vi "בדיקת מתח תפיסה של סליל פיקוד ללא עומס Mod.vi"(8 "error":errorcluster, 9 "מתח מקס":dbl=18.0 format="%#_13g", 10 "שם הממסר":string="0410-24534 15A ממסר", 11 "Path for Log":path) -> (0 "error out":errorcluster, 1 "מצב ממסר פתוח/סגור":bool, 2 "מתח סגירת הממסר":dbl format="%.4f", 3 "מתח מוצא מהספק":dbl format="%.4f", 5 "resultUserPrompt":bool)   [LabVIEW 2014]
uses:
  <vilib>/DAQmx/create/channels.llb/DAQmx Create Channel (DO-Digital Output).vi
  <vilib>/DAQmx/write.llb/DAQmx Write (Digital Bool 1Line 1Point).vi
panel:
  out "progress":dbl(slide) scale=0.0..36.0
  out "error IO DMM":errorcluster
  in  "Stop Button":bool
  # "Right-Click to\nexplain error"
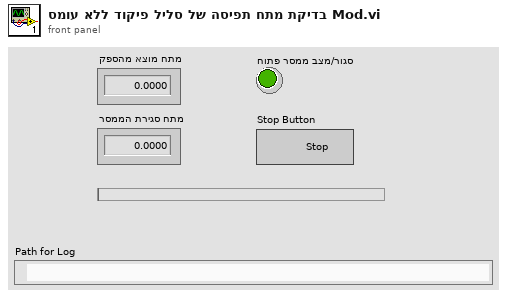
[diagram p1: front panel]
types:
  T1 = enum32{"Invalid", "Standard", "Closed", "Hidden", "Minimized", "Maximized"}
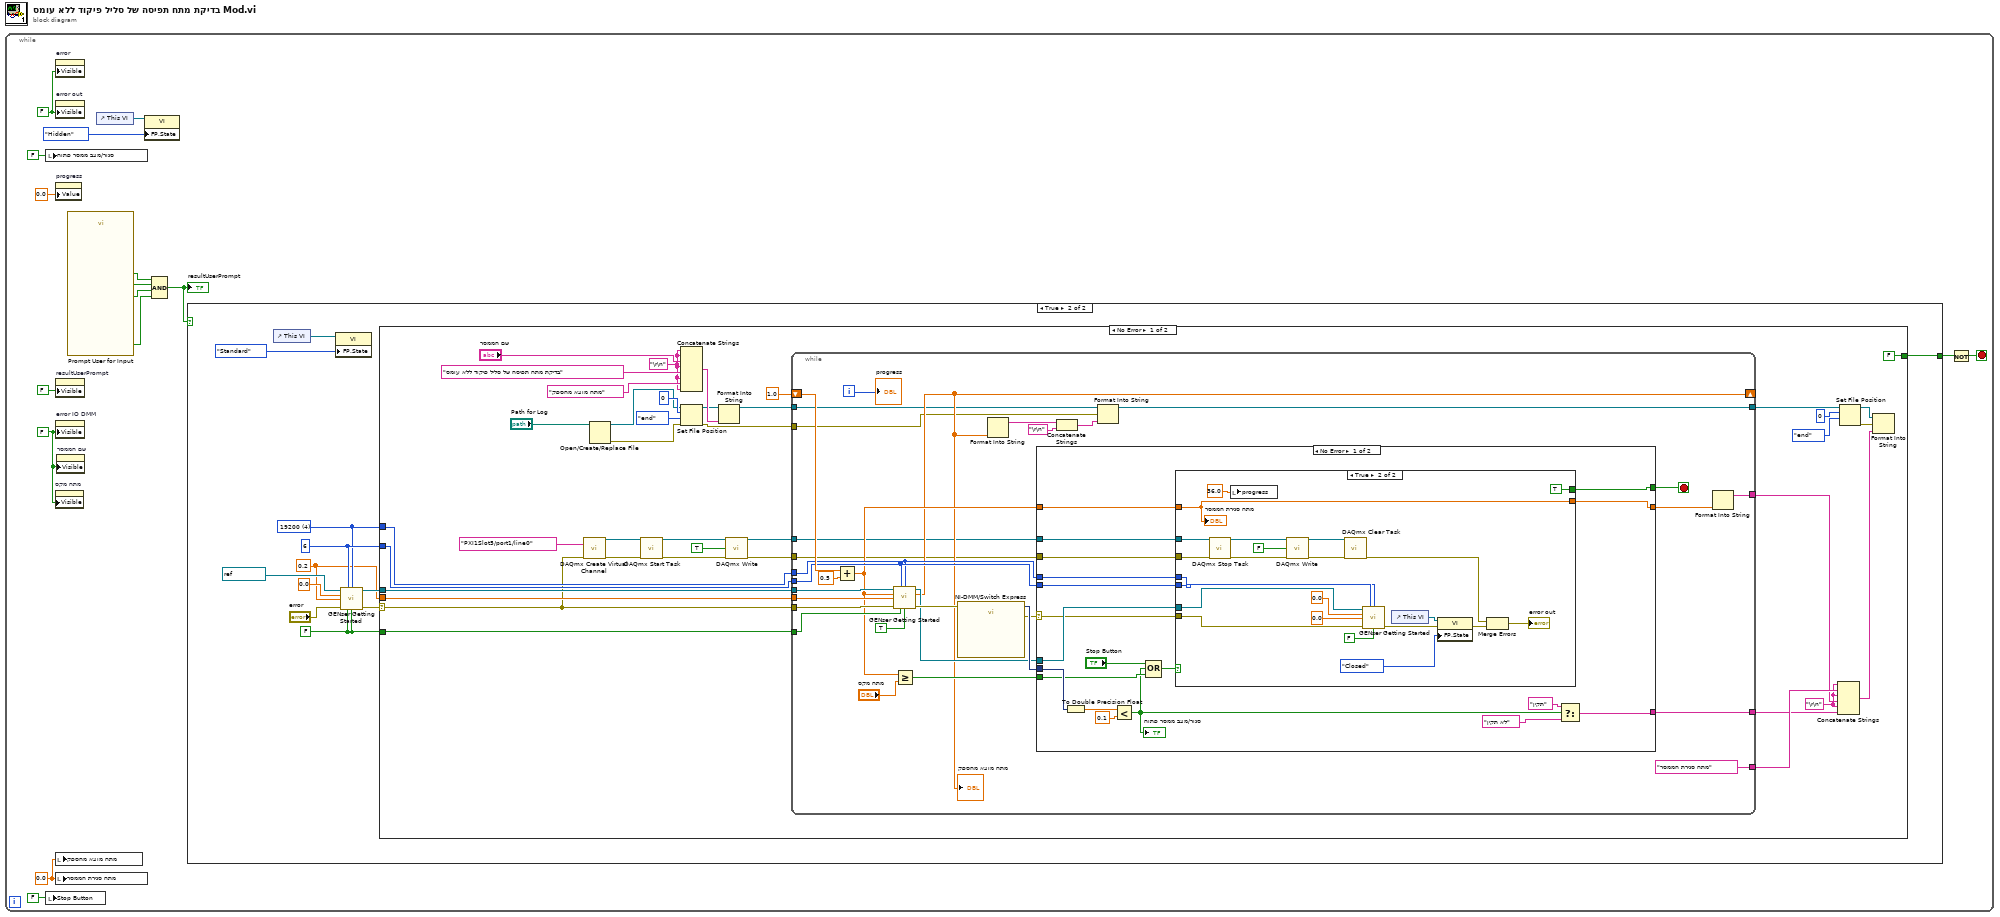
[diagram p0: block diagram]
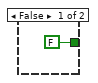
[diagram p2: hidden frame]
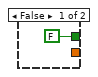
[diagram p3: hidden frame]
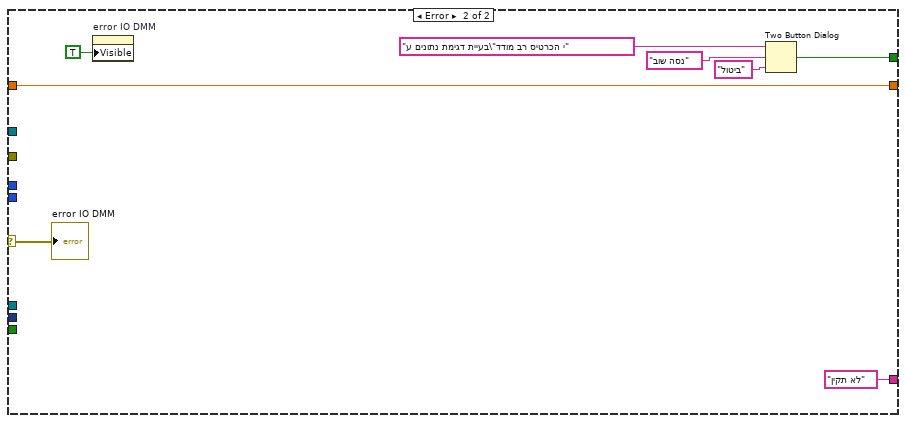
[diagram p4: hidden frame]
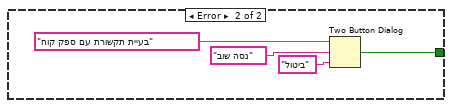
[diagram p5: hidden frame]
diagram:
  n1 = while {
    stop <- w4 stop-if-true
    w3 = FALSE ("Visible")
    w9 = 0.0 ("signals out")
    w1 = FALSE ("Visible")
    n2 = local write "מצב ממסר פתוח/סגור"(FALSE ("מגע סגור")) -> ()
    n3 = local write "Stop Button"(FALSE ("Reset (T)")) -> ()
    n4 = property on="מתח מקס" class="DigNum (strict)"("Visible"=w1) -> ()  [unwired: 2 in, 2 out]
    n5 = property on="error" class="Clust (strict)"("Visible"=w3) -> ()  [unwired: 2 in, 2 out]
    n6 = property on="error out" class="Clust (strict)"("Visible"=w3) -> ()  [unwired: 2 in, 2 out]
    n7 = property on="progress" class="Slide (strict)"("Value"=0.0 ("progress")) -> ()  [unwired: 2 in, 2 out]
    n8 = property on="resultUserPrompt" class="Bool (strict)"("Visible"=FALSE) -> ()  [unwired: 2 in, 2 out]
    n9 = property on="error IO DMM" class="Clust (strict)"("Visible"=w1) -> ()  [unwired: 2 in, 2 out]
    n10 = local write "מתח מוצא מהספק"(w9) -> ()
    n11 = local write "מתח סגירת הממסר"(w9) -> ()
    n12 = property on="שם הממסר" class="Str"("Visible"=w1) -> ()  [unwired: 2 in, 2 out]
    n13 = call "Prompt User for Input"() -> ("הדקי הרב מודד"=w7:bool, "מגע שלילי"=w13:bool, "מגע חיובי"=w14:bool, "OK"=w8:bool)  [unwired: 15 in, 1 out]
    n14 = control-ref of="This VI"() -> (w6:refnum<vi>)
    n15 = property class="VI"(reference=w6, "FP.State"=T1."Hidden" ("Front Panel Window:State")) -> ()  [unwired: 1 in, 2 out]
    n16 = Compound Arithmetic op=AND(w8, w14, w13, w7) -> (w15:bool)
    "resultUserPrompt" <- w15
    n17 = case shown="True" w15 {
      tunnel: [FALSE ("T button?") w23] -> w16
      frame False {
      }
      frame True {
        w22 = FALSE ("Output On (T)")
        w27 = u16 4 items=["1200", "2400", "4800", "9600", "19200"] ("BAUD")
        w28 = i16 6 ("GEN Addr")
        w24 = 0.2 ("Current Limit")
        n18 = control-ref of="This VI"() -> (w20:refnum<vi>)
        n19 = property class="VI"(reference=w20, "FP.State"=T1."Standard" ("Front Panel Window:State")) -> ()  [unwired: 1 in, 2 out]
        n20 = call "GENser Getting Started.vi"("VISA"=refnum<visa-resource-name> "COM6", "GEN Addr"=w28, "BAUD"=w27, "Voltage Limit"=0.0, "Current Limit"=w24, "error"="error", "Reset (T)"=w22, "Output On (T)"=w22) -> ("VISA out"=w29:refnum<visa-resource-name>, "error out"=w19:errorcluster)  [unwired: 4 in, 2 out]
        n21 = case shown="No Error" w19 {
          selector: w19 -> [w30 _]
          tunnel: w29 -> [w68 _]
          tunnel: w28 -> [w67 _]
          tunnel: w27 -> [w66 _]
          tunnel: w22 -> [w65 _]
          tunnel: w24 -> [w64 _]
          tunnel: [FALSE w151] -> w23
          frame No Error {
            w39 = "\r\n"
            w58 = "\r\n"
            n22 = call-poly <vilib>:"DAQmx Create Virtual Channel.vi"("lines"=tag "PXI1Slot5/port1/line0", "error in"=w30) -> ("task out"=w37:refnum<k21>, "error out"=w38:errorcluster)  [unwired: 12 in]
            n23 = Open/Create/Replace File(file path (use dialog)="Path for Log") -> (refnum out=w49:refnum<file>, error out=w48:errorcluster)  [unwired: 5 in, 1 out]
            n24 = call <vilib>:"DAQmx Start Task.vi"("task/channels in"=w37, "error in"=w38) -> ("task out"=w34:refnum<k21>, "error out"=w33:errorcluster)  [unwired: 12 in]
            n25 = Concatenate Strings(w39, w39, "שם הממסר", w39, "בדיקת מתח תפיסה של סליל פיקוד ללא עומס", w39, "מתח מוצא מהספק", w39) -> (w45:string)
            n26 = Set File Position(offset (in bytes) (0)=i64 0, refnum=w49, from (0:start)=enum16{"start", "end", "current"}."end", error in=w48) -> (refnum out=w41:refnum<file>, error out=w46:errorcluster)
            n27 = Format Into String(initial string=w41, w45) -> (resulting string=w40:refnum<file>)  [unwired: 2 in, 1 out]
            n28 = call-poly <vilib>:"DAQmx Write.vi"("task/channels in"=w34, "data"=TRUE, "error in"=w33) -> ("task out"=w32:refnum<k21>, "error out"=w31:errorcluster)  [unwired: 10 in, 1 out]
            n29 = while {
              tunnel: w68 -> [w88]
              tunnel: w30 -> [w99]
              tunnel: w67 -> [w90]
              tunnel: w66 -> [w89]
              tunnel: w65 -> [w98]
              tunnel: w64 -> [w96]
              shift-right: [w80] -> _
              shift-left: 1.0 ("y") -> [w94]
              tunnel: ["מתח סגירת הממסר"] -> w61
              tunnel: [w78] -> w60
              tunnel: [w77] -> w59
              tunnel: [w74] -> w57
              tunnel: w40 -> [w73]
              tunnel: w46 -> [w72]
              tunnel: w32 -> [w70]
              tunnel: w31 -> [w69]
              i -> [w81]
              stop <- w91 stop-if-true
              n30 = Add(x=w94, y=0.5) -> (x+y=w82:dbl)
              n31 = call "GENser Getting Started.vi"("VISA"=w88, "GEN Addr"=w90, "BAUD"=w89, "Voltage Limit"=w82, "Current Limit"=w96, "error"=w99, "Reset (T)"=w98, "Output On (T)"=TRUE) -> ("VISA out"=w87:refnum<visa-resource-name>, "Output Voltage"=w80:dbl, "error out"=w93:errorcluster)  [unwired: 4 in, 1 out]
              "מתח מוצא מהספק" <- w80
              n32 = Greater Or Equal?(x=w82, y="מתח מקס") -> (x >= y?=w85:bool)
              n33 = call "NI-DMM/Switch Express"("error in"=w93) -> ("signals out"=w92:dynamicdata, "error out"=w84:errorcluster)  [unwired: 16 in, 1 out]
              n34 = Format Into String(w80) -> (resulting string=w75:string)  [unwired: 3 in, 1 out]
              n35 = case shown="No Error" w84 {
                selector: w84 -> [w110 w150]
                tunnel: w92 -> [w118 _]
                tunnel: [w107 w146] -> w91
                tunnel: w90 -> [w115 _]
                tunnel: w89 -> [w114 _]
                tunnel: w87 -> [w113 _]
                tunnel: w85 -> [w112 _]
                tunnel: w82 -> [w111 w144]
                tunnel: [w106 w144] -> w83
                tunnel: [w103 "לא תקין"] -> w77
                tunnel: w70 -> [w101 _]
                tunnel: w69 -> [w100 _]
                frame No Error {
                  n36 = To Double Precision Float(number=w118) -> (double precision float=w109:dbl)
                  n37 = Less?(x=w109, y=0.1) -> (x < y?=w102:bool)
                  "מצב ממסר פתוח/סגור" <- w102
                  n38 = Compound Arithmetic op=OR("Stop Button", w102, w112) -> (w117:bool)
                  n39 = case shown="True" w117 {
                    tunnel: [FALSE TRUE] -> w107
                    tunnel: w115 -> [_ w142]
                    tunnel: w114 -> [_ w141]
                    tunnel: w113 -> [_ w140]
                    tunnel: w110 -> [_ w137]
                    tunnel: w111 -> [_ w132]
                    tunnel: [_ w132] -> w106
                    tunnel: w101 -> [_ w122]
                    tunnel: w100 -> [_ w121]
                    frame False {
                    }
                    frame True {
                      n40 = call <vilib>:"DAQmx Stop Task.vi"("task/channels in"=w122, "error in"=w121) -> ("task out"=w130:refnum<k21>, "error out"=w128:errorcluster)  [unwired: 12 in]
                      n41 = local write "progress"(36.0 ("progress")) -> ()
                      n42 = call-poly <vilib>:"DAQmx Write.vi"("task/channels in"=w130, "data"=FALSE, "error in"=w128) -> ("task out"=w127:refnum<k21>, "error out"=w126:errorcluster)  [unwired: 10 in, 1 out]
                      n43 = call <vilib>:"DAQmx Clear Task.vi"("task in"=w127, "error in"=w126) -> ("error out"=w123:errorcluster)  [unwired: 13 in]
                      n44 = call "GENser Getting Started.vi"("VISA"=w140, "GEN Addr"=w142, "BAUD"=w141, "Voltage Limit"=0.0, "Current Limit"=0.0, "error"=w137, "Output On (T)"=FALSE) -> ("error out"=w120:errorcluster)  [unwired: 5 in, 3 out]
                      n45 = control-ref of="This VI"() -> (w134:refnum<vi>)
                      n46 = property class="VI"(reference=w134, error in=w120, "FP.State"=T1."Closed" ("Front Panel Window:State")) -> (error out=w124:errorcluster)  [unwired: 1 out]
                      n47 = Merge Errors(w123, w124) -> (→"error out":errorcluster)
                      "מתח סגירת הממסר" <- w132
                    }
                  }
                  n48 = Select(t="תקין", s=w102, f="לא תקין") -> (s? t:f=w103:string)
                }
                frame Error {
                  n49 = property on="error IO DMM" class="Clust (strict)"("Visible"=TRUE) -> ()  [unwired: 2 in, 2 out]
                  n50 = Two Button Dialog(message="בעיית דגימת נתונים ע\"י הכרטיס רב מודד", 1:"ביטול" ("F button name (\"Cancel\")"), 2:"נסה שוב" ("T button name (\"OK\")")) -> (T button?=w146:bool)
                  "error IO DMM" <- w150
                }
              }
              n51 = Concatenate Strings(w75, "\r\n") -> (w71:string)
              n52 = Format Into String(initial string=w73, error in=w72, w71) -> (resulting string=w74:refnum<file>)  [unwired: 1 in, 1 out]
              n53 = Format Into String(w83) -> (resulting string=w78:string)  [unwired: 3 in, 1 out]
              "progress" <- w81
            }
            n54 = Concatenate Strings(w58, w61, w58, w60, w58, w59) -> (w52:string)
            n55 = Set File Position(offset (in bytes) (0)=i64 0, refnum=w57, from (0:start)=enum16{"start", "end", "current"}."end") -> (refnum out=w54:refnum<file>, error out=w53:errorcluster)  [unwired: 1 in]
            n56 = Format Into String(initial string=w54, error in=w53, w52) -> ()  [unwired: 1 in, 2 out]
          }
          frame Error {
            n57 = Two Button Dialog(message="בעיית תקשורת עם ספק קוח", 1:"ביטול" ("F button name (\"Cancel\")"), 2:"נסה שוב" ("T button name (\"OK\")")) -> (T button?=w151:bool)
          }
        }
      }
    }
    n58 = Not(x=w16) -> (.not. x?=w4:bool)
  }
